vi "_StopSignal-WaitDestroyCompleted.vi"(8 "error in (no error)":errorcluster, 9 "timeout":i32=-1, 11 "Signal Ref":T1) -> (0 "error out":errorcluster)   [LabVIEW 2017, in "StopSignal.lvlib"]
uses:
  StopSignal.lvlib
  Typedef/StopSignal.ctl
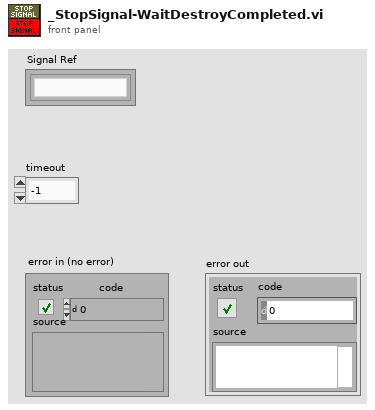
[diagram p1: front panel]
types:
  T1 = typedef "StopSignal.lvlib/StopSignal.ctl" = refnum<k1>
  T2 = typedef "StopSignal.lvlib/_StopSignalData.ctl" = cluster{"StopEvent":refnum<user-event>, "StopNotifier":refnum<notifier>, "StopReason":T3, "DestroyEvent":refnum<user-event>}
  T3 = typedef "StopSignal.lvlib/StopReason.ctl" = cluster{"Reason":string, "timestamp":timestamp}
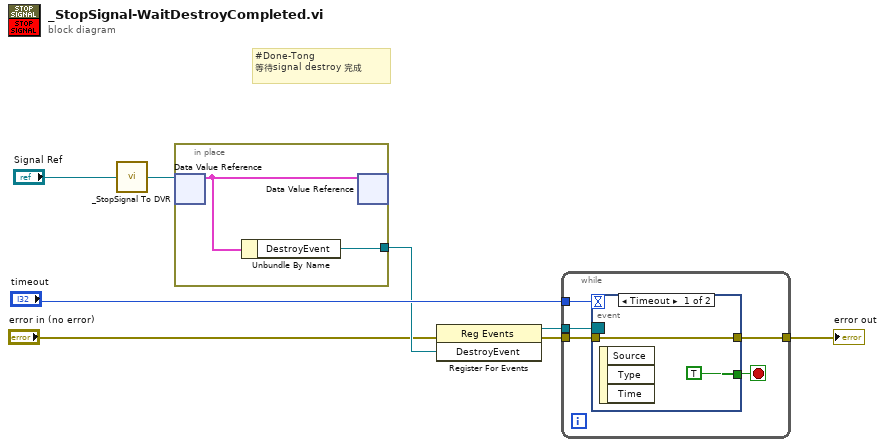
[diagram p0: block diagram]
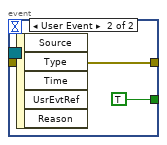
[diagram p2: hidden frame]
diagram:
  # "#Done-Tong\n等待signal destroy 完成"
  n1 = call "_StopSignal To DVR.vi"("Refnum in"="Signal Ref") -> ("Data Value Reference out"=w7:refnum<data-value>)
  n2 = in-place {
    in-place-border: [w9] -> w4
    n3 = in-place-dvr #1(w7) -> (w10:T2)  [unwired: 1 out]
    n4 = Unbundle By Name(w10) -> ("DestroyEvent"=w9:refnum<user-event>)
    n5 = in-place-dvr #1(w10) -> ()  [unwired: 2 out]
  }
  n6 = register-events(error in="error in (no error)", w4) -> (reference out=w6:refnum<event-registration>, error out=w2:errorcluster)  [unwired: 1 in]
  n7 = while {
    tunnel: w6 -> [w15]
    tunnel: "timeout" -> [w13]
    tunnel: w2 -> [w12]
    tunnel: [w11] -> w1
    stop <- w14 stop-if-true
    n8 = event shown="[0] Timeout" {
      selector: w15 -> [_ _]
      dyn-events: _ -> [_ _]
      timeout: w13 -> [_ _]
      tunnel: [TRUE TRUE] -> w14
      tunnel: w12 -> [w16 w18]
      tunnel: [w16 w18] -> w11
      event Timeout {
        n9 = event-data() -> ()  [unwired: 1 in, 3 out]
      }
      event User Event {
        n10 = event-data() -> ()  [unwired: 1 in, 5 out]
      }
    }
  }
  "error out" <- w1
